vi "CreateCommands.vi"   [LabVIEW 2015]
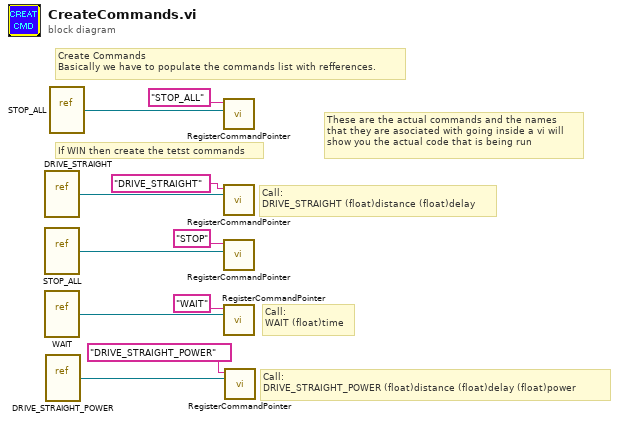
[diagram p0: block diagram]
diagram:
  # "Call:\nDRIVE_STRAIGHT_POWER (float)distance (float)delay (float)power"
  # "Call:\nDRIVE_STRAIGHT (float)distance (float)delay"
  # "These are the actual commands and the names \nthat they are asociated with going inside a vi will\nshow you the actual code that is being run"
  # "Call:\nWAIT (float)time"
  # "If WIN then create the tetst commands"
  # "Create Commands\nBasically we have to populate the commands list with refferences."
  n1 = vi-ref "DRIVE_STRAIGHT.vi"() -> (w7:refnum<vi>)
  n2 = vi-ref "STOP_ALL.vi"() -> (w4:refnum<vi>)
  n3 = vi-ref "WAIT.vi"() -> (w5:refnum<vi>)
  n4 = vi-ref "DRIVE_STRAIGHT_POWER.vi"() -> (w1:refnum<vi>)
  n5 = vi-ref "STOP_ALL.vi"() -> (w9:refnum<vi>)
  n6 = call "RegisterCommandPointer.vi"("Strict-Typed VI Refnum"=w9, "Name"="STOP_ALL") -> ()  [unwired: 10 in]
  n7 = call "RegisterCommandPointer.vi"("Strict-Typed VI Refnum"=w7, "Name"="DRIVE_STRAIGHT") -> ()  [unwired: 10 in]
  n8 = call "RegisterCommandPointer.vi"("Strict-Typed VI Refnum"=w4, "Name"="STOP") -> ()  [unwired: 10 in]
  n9 = call "RegisterCommandPointer.vi"("Strict-Typed VI Refnum"=w5, "Name"="WAIT") -> ()  [unwired: 10 in]
  n10 = call "RegisterCommandPointer.vi"("Strict-Typed VI Refnum"=w1, "Name"="DRIVE_STRAIGHT_POWER") -> ()  [unwired: 10 in]
